vi "Disconnect from Machine.vi"(8 "error in":errorcluster, 11 "Machine In":refnum<visa-resource-name>) -> (0 "error out":errorcluster)   [LabVIEW 2017]
doc: "Closes connection with USB device. \n\n<B>Inputs</B>: \n- Machine In: Specifies the desired machine connected to computer via USB.\n- Firmware: Specifies the machine firmware. Supported firmwares are Grbl and uArm Swift Pro.\n- Error In: reads error (if any) from previous vi."
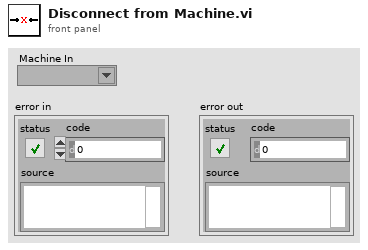
[diagram p1: front panel]
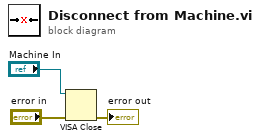
[diagram p0: block diagram]
diagram:
  n1 = VISA Close(VISA resource name="Machine In", error in (no error)="error in") -> (error out=→"error out":errorcluster)
